vi "rs3 Advanced get depth table3.vi"(8 "error in (no error)":errorcluster, 10 "mode":i32, 11 "device in":u64) -> (0 "error out 2":errorcluster, 1 "error":u64, 2 "Depth Table":T1={"depthUnits, um"=1000, "depthClampMin"=0, "depthClampMax"=65000, "disparityMultiplier"=1, "disparityShift"=0}, 3 "Dev out":u64)   [LabVIEW 2017, in "libRealSense3.lvlib"]
doc: "Opens communication to a specific RealSense Device."
uses:
  libRealSense3.lvlib
  realsense2.dll
panel:
  # "RS3 Adv. Get Depth Table3"
  # "(C) 2017 Intel Corp.,  AGJ"
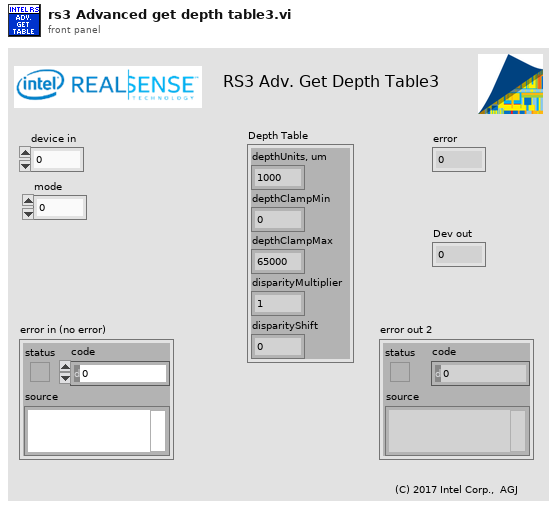
[diagram p1: front panel]
types:
  T1 = cluster{"depthUnits, um":u32, "depthClampMin":u32, "depthClampMax":u32, "disparityMultiplier":u32, "disparityShift":u32}
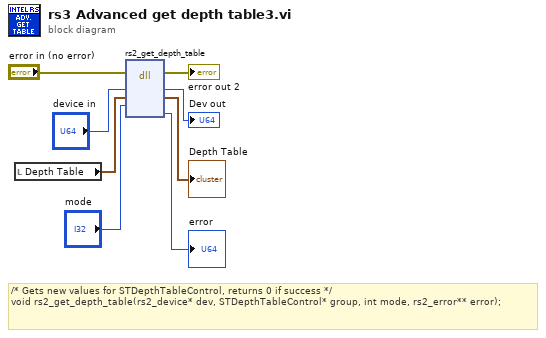
[diagram p0: block diagram]
diagram:
  # "/* Gets new values for STDepthTableControl, returns 0 if success */\nvoid rs2_get_depth_table(rs2_device* dev, STDepthTableControl* group, int mode, rs2_error** error);"
  n1 = local read "Depth Table"() -> (w4:T1)
  n2 = dll-call lib="C:/Users/agrunnet/Documents/libRealSense6/realsense2.dll" fn="rs2_get_depth_table"(error in="error in (no error)", "device"="device in", "depth control"=w4, "mode"="mode") -> (error out=→"error out 2":errorcluster, "device"=→"Dev out":u64, "depth control"=→"Depth Table":T1, "error"=→"error":u64)  [unwired: 5 in, 1 out]
